vi "Call_signal_fromfile.vi"(6 "Plot window":string) -> (0 "Y subarray":string[](array[string]), 1 "X subarray":string[](array[string]), 2 "Curve name":string(combo), 3 "Ready?":bool)   [LabVIEW 2022 SP3]
doc: "Through this function you can select the signals stored in a CSV file."
uses:
  <vilib>/Utility/file.llb/Read Delimited Spreadsheet (string).vi
panel:
  out "Clone Name":string
  in  "Close app":bool
  in  "X data":string(combo)
  out "all rows":string[][](array[string])
  in  "Y data":string(combo)
  in  "Add":bool
  in  "Cancel":bool
  in  "From file (csv)":path caption="file path (dialog if empty)"
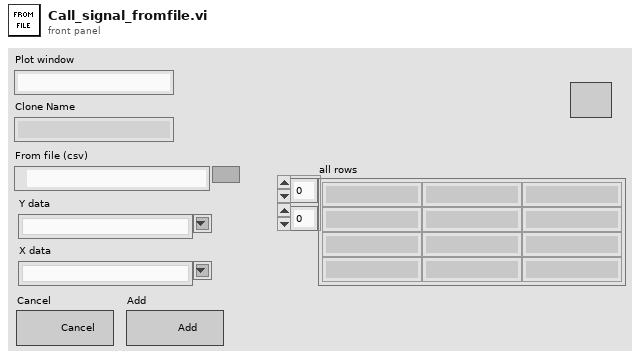
[diagram p1: front panel]
types:
  T1 = enum32{"Invalid", "Standard", "Closed", "Hidden", "Minimized", "Maximized"}
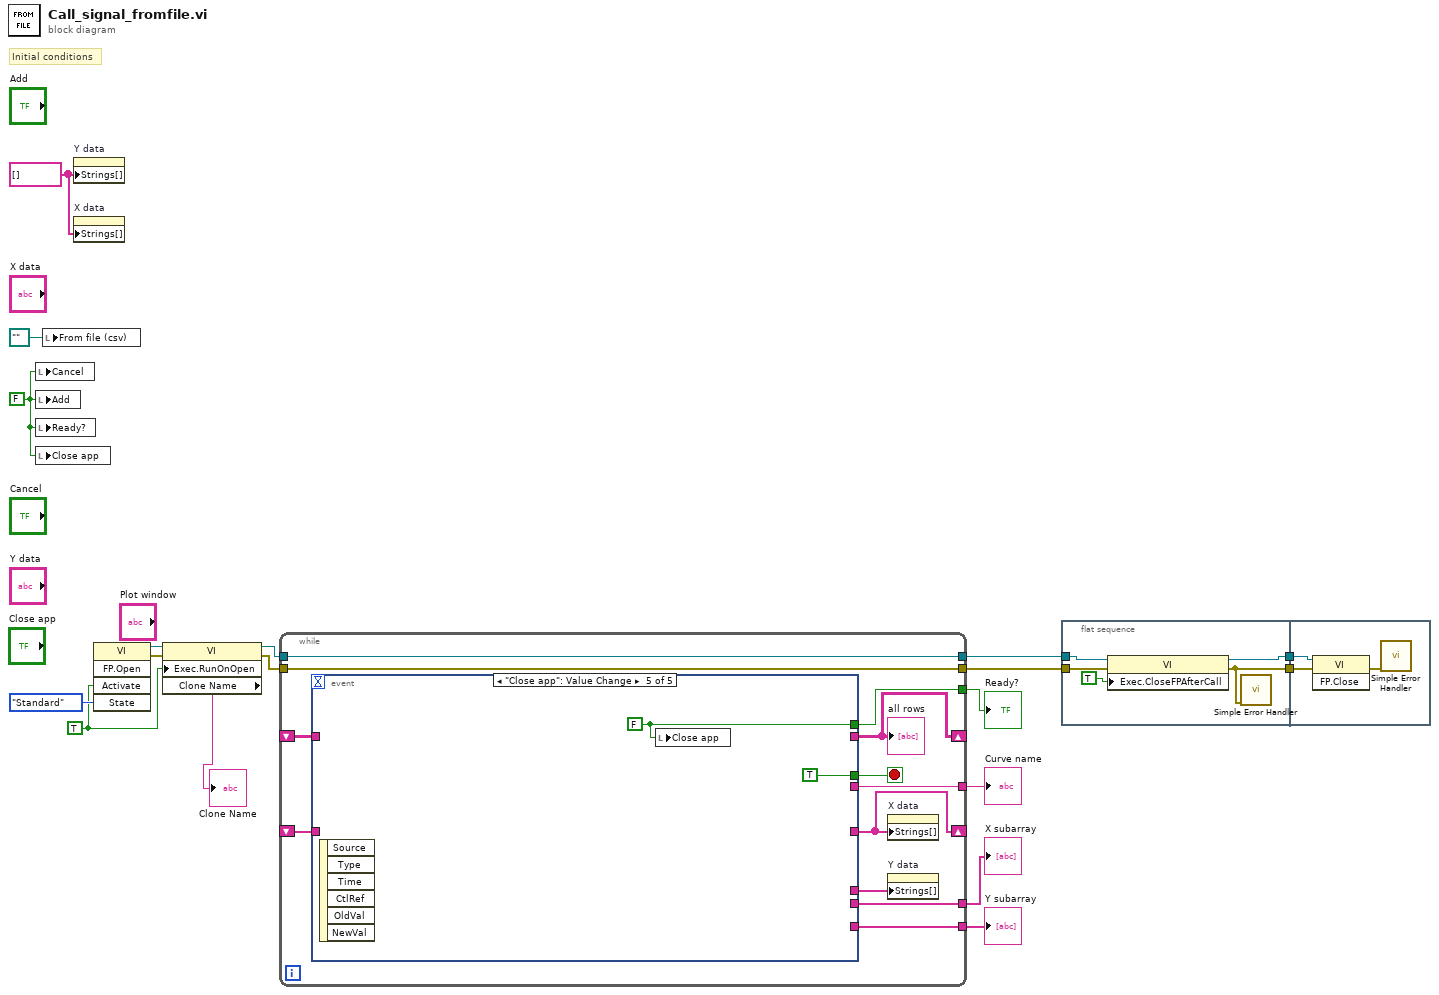
[diagram p0: block diagram]
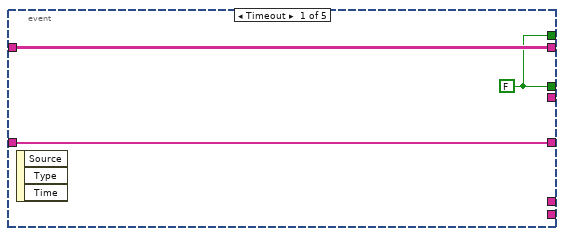
[diagram p2: hidden frame]
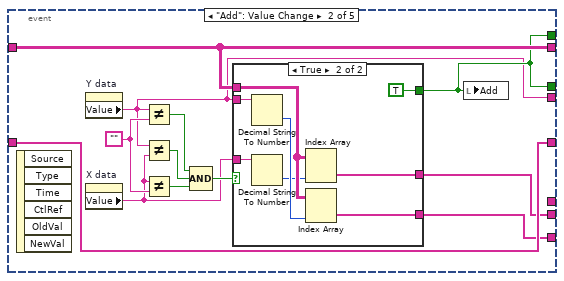
[diagram p3: hidden frame]
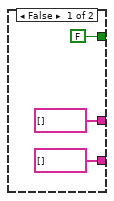
[diagram p4: hidden frame]
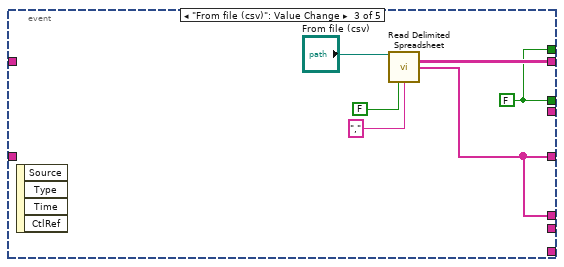
[diagram p5: hidden frame]
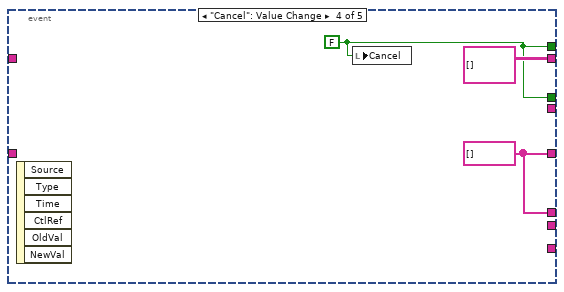
[diagram p6: hidden frame]
diagram:
  w9 = TRUE ("Activate?")
  w4 = string[] [] ("Strings []")
  w2 = FALSE
  # "Initial conditions"
  n1 = local write "Cancel"(w2) -> ()
  n2 = local write "Add"(w2) -> ()
  n3 = local write "Ready?"(w2) -> ()
  n4 = local write "Close app"(w2) -> ()
  n5 = local write "From file (csv)"(path "" ("From file (csv)")) -> ()
  n6 = property on="Y data" class="CmbBox"("Strings[]"=w4) -> ()  [unwired: 2 in, 2 out]
  n7 = property on="X data" class="CmbBox"("Strings[]"=w4) -> ()  [unwired: 2 in, 2 out]
  n8 = invoke class="VI" method="FP.Open"("Activate"=w9, "State"=T1."Standard") -> (reference out=w11:refnum<vi>, error out=w12:errorcluster)  [unwired: 3 in, 3 out]
  n9 = property class="VI"(reference=w11, error in=w12, "Exec.RunOnOpen"=w9) -> (reference out=w10:refnum<vi>, error out=w13:errorcluster, "Clone Name"=→"Clone Name":string)
  n10 = while {
    shift-right: [w27] -> _
    shift-left: _ -> [w29]
    shift-right: [w22] -> _
    shift-left: _ -> [w28]
    tunnel: [w26] -> w17
    tunnel: [w25] -> w16
    tunnel: [w23] -> w15
    tunnel: w13 -> [w20]
    tunnel: w10 -> [w21]
    tunnel: [w21] -> w8
    tunnel: [w20] -> w7
    tunnel: [w19] -> w3
    stop <- w30 stop-if-true
    n11 = event shown="[4] \"Close app\": Value Change" {
      selector: _ -> [_ _ _ _ _]
      dyn-events: _ -> [_ _ _ _ _]
      timeout: _ -> [_ _ _ _ _]
      tunnel: [w33 w40 w59 string[][] [] ("all rows") _] -> w27
      tunnel: [w32 w39 w58 w64 _] -> w22
      tunnel: [w31 w35 w57 w63 TRUE] -> w30
      tunnel: w29 -> [w33 w40 _ _ _]
      tunnel: w28 -> [w32 w39 _ _ _]
      tunnel: [_ w38 _ _ _] -> w26
      tunnel: [_ w37 _ _ _] -> w25
      tunnel: [_ _ w58 w64 _] -> w24
      tunnel: [w31 w35 w57 w63 w66] -> w23
      tunnel: [_ w34 _ _ _] -> w19
      event Timeout {
        w31 = FALSE
        n12 = event-data() -> ()  [unwired: 1 in, 3 out]
      }
      event "Add": Value Change {
        w42 = ""
        n13 = event-data() -> ()  [unwired: 1 in, 6 out]
        n14 = property on="Y data" class="CmbBox"() -> ("Value"=w34:string)  [unwired: 2 in, 2 out]
        n15 = property on="X data" class="CmbBox"() -> ("Value"=w36:string)  [unwired: 2 in, 2 out]
        n16 = Not Equal?(x=w34, y=w42) -> (x != y?=w43:bool)
        n17 = Not Equal?(x=w34, y=w36) -> (x != y?=w44:bool)
        n18 = Not Equal?(x=w36, y=w42) -> (x != y?=w45:bool)
        n19 = Compound Arithmetic op=AND(w43, w44, w45) -> (w41:bool)
        n20 = case shown="True" w41 {
          tunnel: [FALSE TRUE] -> w35
          tunnel: w40 -> [_ w53]
          tunnel: w34 -> [_ w55]
          tunnel: w36 -> [_ w52]
          tunnel: [string[] [] ("all rows") w50] -> w38
          tunnel: [string[] [] ("all rows") w49] -> w37
          frame False {
          }
          frame True {
            n21 = Decimal String To Number(string=w55) -> (number=w54:i32)  [unwired: 2 in, 1 out]
            n22 = Decimal String To Number(string=w52) -> (number=w51:i32)  [unwired: 2 in, 1 out]
            n23 = Index Array(array=w53, index (col)=w51) -> (element=w49:string[])  [unwired: 1 in]
            n24 = Index Array(array=w53, index (col)=w54) -> (element=w50:string[])  [unwired: 1 in]
          }
        }
        n25 = local write "Add"(w35) -> ()
      }
      event "From file (csv)": Value Change {
        w57 = FALSE
        n26 = event-data() -> ()  [unwired: 1 in, 4 out]
        n27 = call-poly <vilib>:"Read Delimited Spreadsheet.vi"("file path (dialog if empty)"="From file (csv)", "transpose? (F)"=FALSE, "delimiter (\\t)"="," ("delimiter (\\t)")) -> ("all rows"=w59:string[][], "first row"=w58:string[])  [unwired: 7 in, 4 out]
      }
      event "Cancel": Value Change {
        w63 = FALSE
        w64 = string[] [] ("first row")
        n28 = event-data() -> ()  [unwired: 1 in, 6 out]
        n29 = local write "Cancel"(w63) -> ()
      }
      event "Close app": Value Change {
        w66 = FALSE
        n30 = event-data() -> ()  [unwired: 1 in, 6 out]
        n31 = local write "Close app"(w66) -> ()
      }
    }
    "all rows" <- w27
    n32 = property on="X data" class="CmbBox"("Strings[]"=w22) -> ()  [unwired: 2 in, 2 out]
    n33 = property on="Y data" class="CmbBox"("Strings[]"=w24) -> ()  [unwired: 2 in, 2 out]
  }
  "Y subarray" <- w17
  "X subarray" <- w16
  "Ready?" <- w15
  "Curve name" <- w3
  n34 = flat-sequence {
    tunnel: w8 -> [w72]
    tunnel: w7 -> [w71]
    tunnel: [w69] -> w6
    tunnel: [w68] -> w5
    tunnel: w6 -> [w74]
    tunnel: w5 -> [w73]
    frame #0 {
      n35 = property class="VI"(reference=w72, error in=w71, "Exec.CloseFPAfterCall"=TRUE ("Activate?")) -> (reference out=w69:refnum<vi>, error out=w68:errorcluster)
      n36 = call <vilib>:"Simple Error Handler.vi"("error in (no error)"=w68) -> ()  [unwired: 4 in, 5 out]
    }
    frame #1 {
      n37 = invoke class="VI" method="FP.Close"(reference=w74, error in=w73) -> (error out=w75:errorcluster)  [unwired: 1 in, 2 out]
      n38 = call <vilib>:"Simple Error Handler.vi"("error in (no error)"=w75) -> ()  [unwired: 4 in, 5 out]
    }
  }
